vi "bmd101ParserQueue.vi"() -> ()   [LabVIEW 2016]
doc: "This example performs writes and reads on a serial port, as directed by the user. You can press the Write and Read buttons, and change the Read Count, while the example is running.\n\nThe parameters set for the serial port must match the parameters of the connected instrument or device. In this example, the Read Count parameter specifies the number of bytes that the serial port reads. If there were more bytes at the port than the specified number, those bytes would not be read. If there were less bytes at the port than the specified number, you would receive a timeout error.\n\nThis example expands upon the flow control options for XON and XOFF, allowing the user to choose those control characters. Also, the user can enable or disable a termination character. Some devices require a termination character in order to identify the end of command strings. Some devices send a termination character to signify the end of data to be read. This example shows how you can end the Read operation once a termination character is detected in the buffer and/or append a termination character at the end of the Write data."
uses:
  C:/Program Files/National Instruments/LabVIEW 2016/examples/Instrument IO/Serial/support/Serial - Settings.ctl
  <vilib>/Instr/_visa.llb/VISA Configure Serial Port (Instr).vi
panel:
  out "return count":u32
  out "Hex String":string[](array[string])
  out "Response":string
  in  "Read Count":u32=1000
  in  "Read":bool=TRUE
  in  "Stop":bool
  in  "Serial Settings":T1={"baud rate"=57600, "data bits"=8, "parity"=enum."None", "stop bits"=10, "flow control"=0} {"flow control" items=["None"=0, "XON/XOFF"=1, "RTS/CTS"=2, "DTR/DSR"=4]; "stop bits" items=["1.0"=10, "1.5"=15, "2.0"=20]; "data bits" min=5 max=8 step=1; "baud rate" items=["75"=75, "110"=110, "134"=134, "150"=150, "300"=300, "600"=600, "1200"=1200, "1800"=1800, "2400"=2400, "4800"=4800, "7200"=7200, "9600"=9600, "14400"=14400, "19200"=19200, "28800"=28800, "38400"=38400, "56000"=56000, "57600"=57600, "115200"=115200, "128000"=128000, "230400"=230400]}
  in  "VISA resource name":refnum<visa-resource-name>="bmd101"
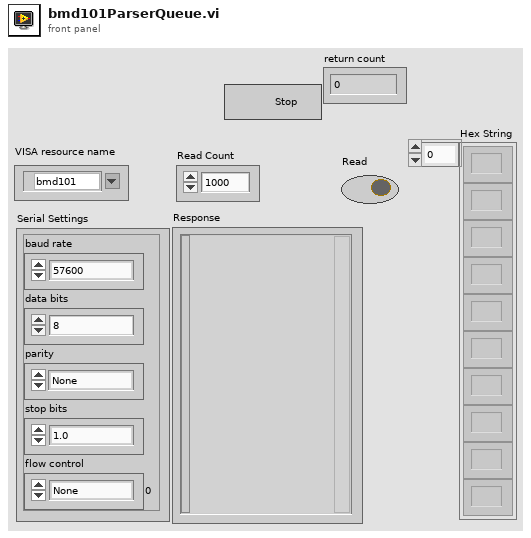
[diagram p1: front panel]
types:
  T1 = typedef "Serial - Settings.ctl" = cluster{"baud rate":u32, "data bits":u16, "parity":enum16{"None", "Odd", "Even", "Mark", "Space"}, "stop bits":u16, "flow control":u16}
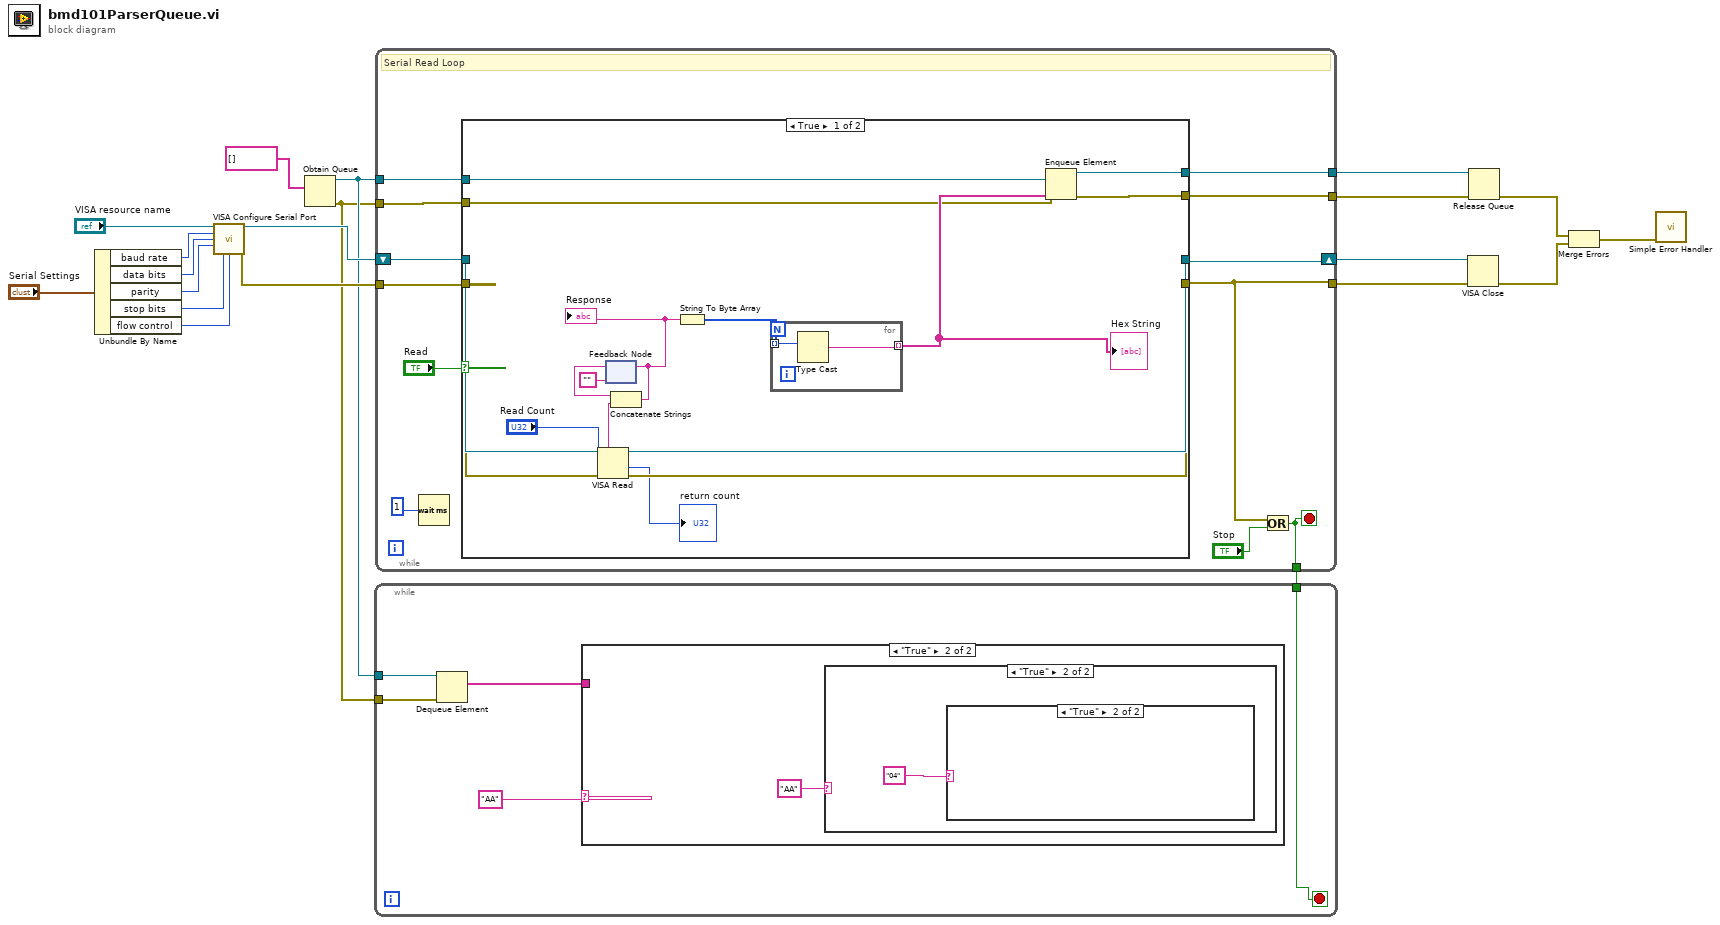
[diagram p0: block diagram]
diagram:
  n1 = Unbundle By Name("Serial Settings") -> ("baud rate"=w19:u32, "data bits"=w18:u16, "parity"=w17:enum16{"None", "Odd", "Even", "Mark", "Space"}, "stop bits"=w16:u16, "flow control"=w15:u16)
  n2 = call-poly "VISA Configure Serial Port"("VISA resource name"="VISA resource name", "baud rate (9600)"=w19, "data bits (8)"=w18, "parity (0:none)"=w17, "stop bits (10: 1 bit)"=w16, "flow control (0:none)"=w15) -> ("VISA resource name out"=w11:refnum<visa-resource-name>, "error out"=w10:errorcluster)  [unwired: 4 in, 4 out]
  n3 = Obtain Queue(element data type=string[] []) -> (queue out=w3:refnum<queue>, error out=w2:errorcluster)  [unwired: 4 in, 1 out]
  n4 = while {
    shift-right: [w32] -> w12
    shift-left: w11 -> [w27]
    tunnel: w10 -> [w26]
    tunnel: [w29] -> w13
    tunnel: w2 -> [w25]
    tunnel: w3 -> [w24]
    tunnel: [w23] -> w8
    tunnel: [w22] -> w7
    tunnel: [w21] -> w1
    stop <- w21 stop-if-true
    # "Serial Read Loop"
    n5 = Wait (ms)(milliseconds to wait=u32 1) -> ()  [unwired: 1 out]
    n6 = case shown="True" "Read" {
      tunnel: [w46 w54] -> w32
      tunnel: w27 -> [w48 w54]
      tunnel: [w44 w53] -> w29
      tunnel: w26 -> [w47 w53]
      tunnel: w25 -> [w35 w51]
      tunnel: w24 -> [w37 w52]
      tunnel: [w36 w52] -> w23
      tunnel: [w34 w51] -> w22
      frame True {
        n7 = VISA Read(VISA resource name=w48, byte count="Read Count", error in (no error)=w47) -> (VISA resource name out=w46:refnum<visa-resource-name>, read buffer=w43:string, return count=→"return count":u32, error out=w44:errorcluster)
        n8 = feedback #1("") -> (w42:string)
        n9 = Concatenate Strings(w42, w43) -> (w39:string)
        "Response" <- w39
        n10 = feedback-in #1(w39) -> ()
        n11 = String To Byte Array(string=w39) -> (unsigned byte array=w40:u8[])
        n12 = for {
          tunnel: w40 -> [w50] mode=indexing
          tunnel: [w49] -> w38 mode=indexing
          n13 = Type Cast(x=w50) -> (*(type *) &x=w49:string)  [unwired: 1 in]
        }
        "Hex String" <- w38
        n14 = Enqueue Element(queue=w37, element=w38, error in (no error)=w35) -> (queue out=w36:refnum<queue>, error out=w34:errorcluster)  [unwired: 1 in, 1 out]
      }
      frame False {
      }
    }
    n15 = Or(x=w29, y="Stop") -> (x .or. y?=w21:bool)
  }
  n16 = while {
    tunnel: w3 -> [w58]
    tunnel: w2 -> [w57]
    tunnel: w1 -> [w55]
    stop <- w55 stop-if-true
    n17 = Dequeue Element(queue=w58, error in (no error)=w57) -> (element=w56:string[])  [unwired: 1 in, 3 out]
    n18 = case shown="\"True\"" "AA" {
      tunnel: w56 -> [_ _]
      frame "False", Default {
      }
      frame "True" {
        n19 = case shown="\"True\"" "AA" {
          frame "False", Default {
          }
          frame "True" {
            n20 = case shown="\"True\"" "04" {
              frame "False", Default {
              }
              frame "True" {
              }
            }
          }
        }
      }
    }
  }
  n21 = VISA Close(VISA resource name=w12, error in (no error)=w13) -> (error out=w4:errorcluster)
  n22 = Release Queue(queue=w8, error in (no error)=w7) -> (error out=w6:errorcluster)  [unwired: 1 in, 2 out]
  n23 = Merge Errors(w6, w4) -> (w5:errorcluster)
  n24 = call <vilib>:"Simple Error Handler.vi"("error in (no error)"=w5) -> ()  [unwired: 1 in, 8 out]
